vi "Session Data.vi"(8 "error in (no error)":errorcluster, 9 "User Data In":T1 {"SMARTDAC+ Type (0: Unknown)" items=["Unknown", "GX10", "GX20", "GP10", "GP20", "GM10"]; "Serial Auth Type (0: Not Auth)" items=["Not Auth", "RS-232C", "RS-422/485", "Bluetooth"]}, 10 "Action (0 : Read Data)":i32(ring) items=["Read Data", "Write Data", "Clear Data", "Clear All Data"], 11 "VISA resource name":refnum<visa-resource-name>) -> (0 "error out":errorcluster, 2 "User Data Out":T1 {"SMARTDAC+ Type (0: Unknown)" items=["Unknown", "GX10", "GX20", "GP10", "GP20", "GM10"]; "Serial Auth Type (0: Not Auth)" items=["Not Auth", "RS-232C", "RS-422/485", "Bluetooth"]}, 3 "VISA resource name out":refnum<visa-resource-name>)   [LabVIEW 2020, in "Yokogawa GX Series.lvlib"]
doc: "This VI logouts from the instrument. Then it can not re-login."
uses:
  <instrlib>/Yokogawa GX Series/Yokogawa GX Series.lvlib
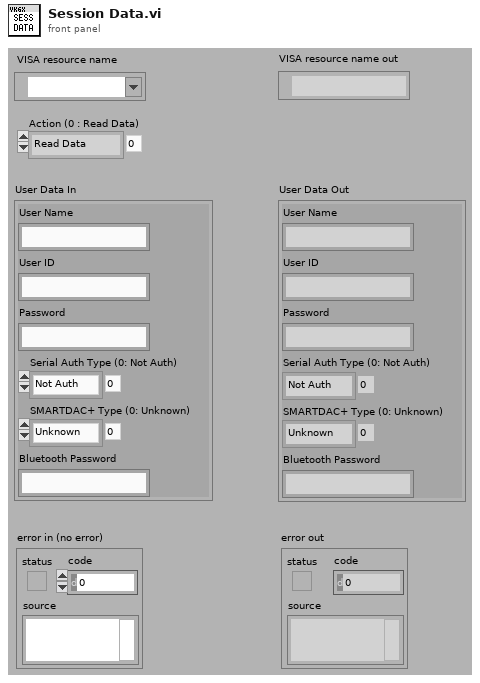
[diagram p1: front panel]
types:
  T1 = cluster{"User Name":string, "User ID":string, "Password":string, "Serial Auth Type (0: Not Auth)":u16, "SMARTDAC+ Type (0: Unknown)":u16, "Bluetooth Password":string}
  T2 = cluster{"User Name":string, "User ID":string, "Password":string, "Serial Auth Type (0: Not Auth)":u16, "SMARTDAC+ Type (0: Unknown)":u16, "Bluetooth Password":string}[]
  T3 = cluster{string, string, string, u16, u16, string}
  T4 = cluster{string, string, string, u16, u16, string}[]
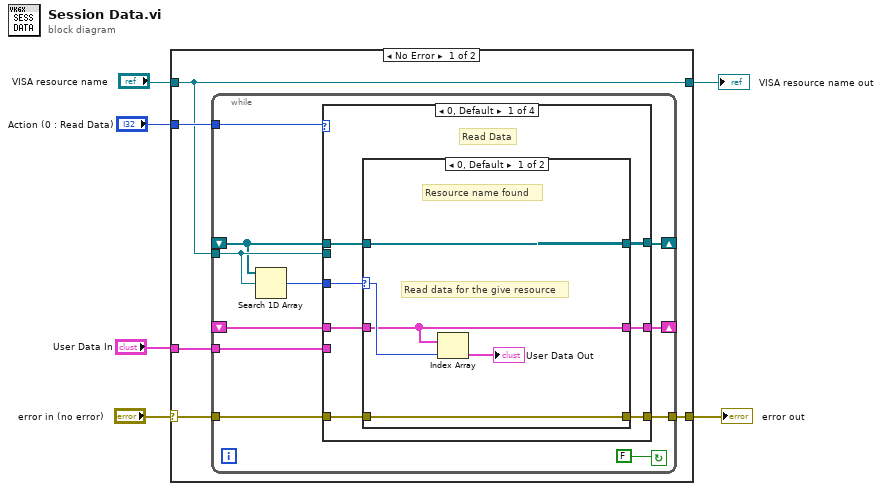
[diagram p0: block diagram]
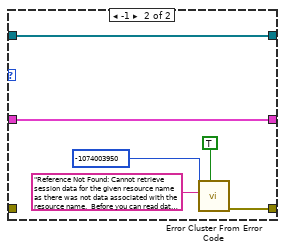
[diagram p2: hidden frame]
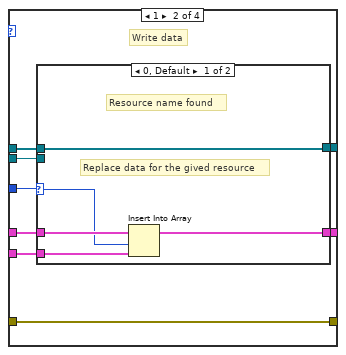
[diagram p3: hidden frame]
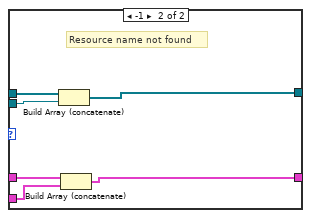
[diagram p4: hidden frame]
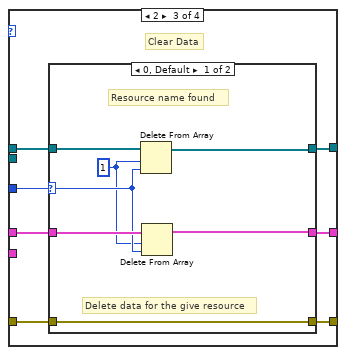
[diagram p5: hidden frame]
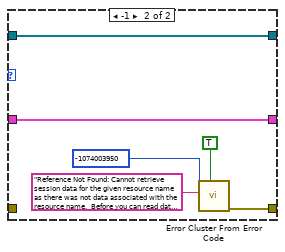
[diagram p6: hidden frame]
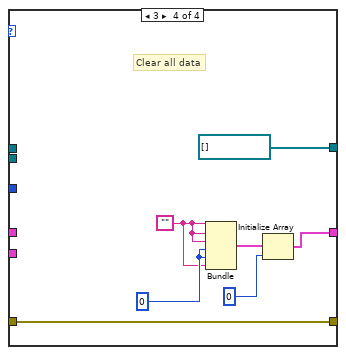
[diagram p7: hidden frame]
diagram:
  n1 = case shown="No Error" "error in (no error)" {
    selector: "error in (no error)" -> [w8 w87]
    tunnel: "VISA resource name" -> [w10 w88]
    tunnel: [w10 w88] -> w5
    tunnel: [w7 w87] -> w4
    tunnel: "Action (0 : Read Data)" -> [w11 _]
    tunnel: "User Data In" -> [w9 _]
    frame No Error {
      n2 = while {
        tunnel: w11 -> [w21]
        tunnel: w10 -> [w20]
        shift-right: [w18] -> _
        shift-left: _ -> [w12]
        tunnel: w9 -> [w15]
        tunnel: w8 -> [w17]
        tunnel: [w16] -> w7
        shift-right: [w14] -> _
        shift-left: _ -> [w13]
        stop <- FALSE continue-if-true
        n3 = Search 1D Array(1D array=w12, element=w20) -> (index of element=w19:i32)  [unwired: 1 in]
        n4 = case shown="0, Default" w21 {
          tunnel: w20 -> [_ w47 _ _]
          tunnel: w19 -> [w29 w48 w66 _]
          tunnel: [w27 w46 w64 refnum<visa-resource-name>[] []] -> w18
          tunnel: w12 -> [w28 w45 w65 _]
          tunnel: w17 -> [w24 w44 w61 w85]
          tunnel: [w23 w44 w60 w85] -> w16
          tunnel: w15 -> [_ w43 _ _]
          tunnel: [w25 w42 w62 w81] -> w14
          tunnel: w13 -> [w26 w41 w63 _]
          frame 0, Default {
            # "Read Data"
            n5 = case shown="0, Default" w29 {
              selector: w29 -> [w33 _]
              tunnel: w28 -> [w34 w40]
              tunnel: [w34 w40] -> w27
              tunnel: w26 -> [w32 w35]
              tunnel: [w32 w35] -> w25
              tunnel: w24 -> [w31 _]
              tunnel: [w31 w36] -> w23
              frame 0, Default {
                # "Read data for the give resource"
                # "Resource name found"
                n6 = Index Array(array=w32, index=w33) -> (element=→"User Data Out":T1)
              }
              frame -1 {
                n7 = call <vilib>:"Error Cluster From Error Code.vi"("show call chain? (False)"=TRUE, "error message (\"\")"="Reference Not Found: Cannot retrieve session data for the given resource name as there was not data associated with the resource name.  Before you can read data, you need to write the session data using the Write Data action of this Session Data VI. ", "error code (0)"=-1074003950) -> ("error out"=w36:errorcluster)  [unwired: 6 in]
              }
            }
          }
          frame 1 {
            # "Write data"
            n8 = case shown="0, Default" w48 {
              selector: w48 -> [w50 _]
              tunnel: w47 -> [_ w59]
              tunnel: [w53 w58] -> w46
              tunnel: w45 -> [w53 w57]
              tunnel: w43 -> [w51 w56]
              tunnel: [w49 w55] -> w42
              tunnel: w41 -> [w52 w54]
              frame 0, Default {
                # "Replace data for the gived resource"
                # "Resource name found"
                n9 = Insert Into Array(array=w52, index=w50, new element=w51) -> (w49:T2)
              }
              frame -1 {
                # "Resource name not found"
                n10 = Build Array (concatenate)(w57, w59) -> (w58:refnum<visa-resource-name>[])
                n11 = Build Array (concatenate)(w54, w56) -> (w55:T2)
              }
            }
          }
          frame 2 {
            # "Clear Data"
            n12 = case shown="0, Default" w66 {
              selector: w66 -> [w68 _]
              tunnel: w65 -> [w72 w79]
              tunnel: [w71 w79] -> w64
              tunnel: w63 -> [w70 w74]
              tunnel: [w69 w74] -> w62
              tunnel: w61 -> [w73 _]
              tunnel: [w73 w75] -> w60
              frame 0, Default {
                w67 = 1
                # "Delete data for the give resource"
                # "Resource name found"
                n13 = Delete From Array(array=w72, length=w67, index=w68) -> (array with subset deleted=w71:refnum<visa-resource-name>[])  [unwired: 1 out]
                n14 = Delete From Array(array=w70, length=w67, index=w68) -> (array with subset deleted=w69:T2)  [unwired: 1 out]
              }
              frame -1 {
                n15 = call <vilib>:"Error Cluster From Error Code.vi"("show call chain? (False)"=TRUE, "error message (\"\")"="Reference Not Found: Cannot retrieve session data for the given resource name as there was not data associated with the resource name.  Before you can read data, you need to write the session data using the Write Data action of this Session Data VI. ", "error code (0)"=-1074003950) -> ("error out"=w75:errorcluster)  [unwired: 6 in]
              }
            }
          }
          frame 3 {
            w82 = u16 0
            w80 = ""
            # "Clear all data"
            n16 = Bundle(w80, w80, w80, w82, w82, w80) -> (w84:T3)  [unwired: 1 in]
            n17 = Initialize Array(w84, 0) -> (w81:T4)
          }
        }
      }
    }
    frame Error {
    }
  }
  "error out" <- w4
  "VISA resource name out" <- w5
